vi "get_next_states.vi"(10 "state":i32[](array[numeric])=[8, 0, 0]) -> (2 "next states":i32[][](array[numeric]))   [LabVIEW 2021]
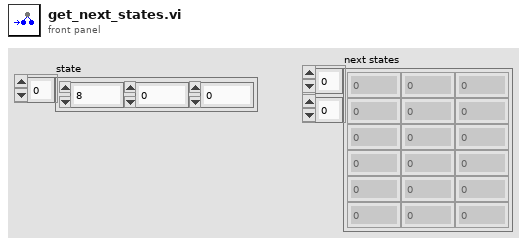
[diagram p1: front panel]
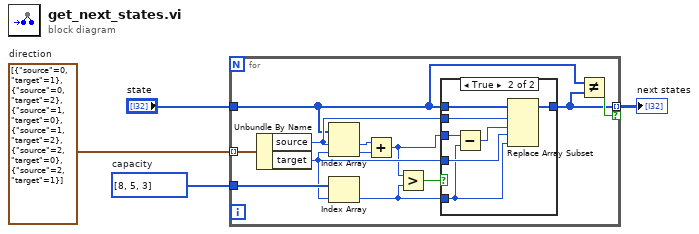
[diagram p0: block diagram]
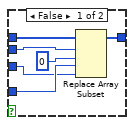
[diagram p2: hidden frame]
diagram:
  w4 = cluster{"source":i32, "target":i32}[] [{"source"=0, "target"=1}, {"source"=0, "target"=2}, {"source"=1, "target"=0}, {"source"=1, "target"=2}, {"source"=2, "target"=0}, {"source"=2, "target"=1}]  # direction
  w2 = i32[] [8, 5, 3]  # capacity
  n1 = for {
    tunnel: w4 -> [w16] mode=indexing
    tunnel: "state" -> [w6]
    tunnel: w2 -> [w14]
    tunnel: [w5] -> w1 mode=indexing if=w7
    n2 = Unbundle By Name(w16) -> ("source"=w12:i32, "target"=w11:i32)
    n3 = Index Array(array=w6, index #1=w12, index #2=w11) -> (element #1=w9:i32, element #2=w15:i32)
    n4 = Index Array(array=w14, index=w11) -> (element=w10:i32)
    n5 = Add(x=w9, y=w15) -> (x+y=w8:i32)
    n6 = Greater?(x=w8, y=w10) -> (0:w13:bool)
    n7 = case shown="True" w13 {
      tunnel: w6 -> [w20 w29]
      tunnel: w12 -> [w22 w28]
      tunnel: w11 -> [w21 w27]
      tunnel: w10 -> [_ w25]
      tunnel: w8 -> [w18 w26]
      tunnel: [w17 w23] -> w5
      frame False {
        n8 = Replace Array Subset(array=w20, new element #1=0 ("new element/subarray"), index #1=w22, new element #2=w18, index #2=w21) -> (w17:i32[])
      }
      frame True {
        n9 = Subtract(x=w26, y=w25) -> (x-y=w24:i32)
        n10 = Replace Array Subset(array=w29, new element #1=w24, index #1=w28, new element #2=w25, index #2=w27) -> (w23:i32[])
      }
    }
    n11 = Not Equal?(x=w6, y=w5) -> (x != y?=w7:bool)
  }
  "next states" <- w1
